vi "Main Monitor Loop.vi"(8 "error in (no error)":errorcluster, 11 "main ref":T1) -> (0 "error out":errorcluster)   [LabVIEW 2025]
uses:
  controls/LAB-IQ UI Data.ctl
  Traction Loop/Traction Receipe Enum.ctl
panel:
  out "Test Stop Temp":bool
  out "DepthZ":dbl
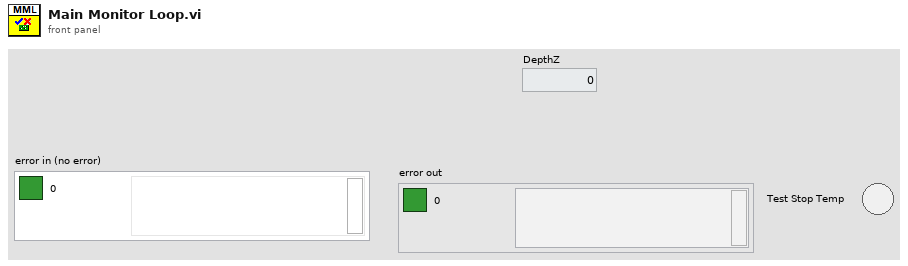
[diagram p1: front panel]
types:
  T1 = typedef "LAB-IQ UI Data.ctl" = cluster{"Main Home Screen":cluster{"GUI":refnum<vi>, "Platform Settings":refnum<vi>, "Configure":refnum<vi>, "Home":refnum<vi>, "EXIT":refnum<vi>, "service 2":refnum<vi>, "MainPage":refnum<vi>, "Analysis":refnum<vi>}, "Platform Settings":cluster{"mm/s  Surge":refnum<vi>, "Update Surge Speed":refnum<vi>, "Drive Error":refnum<vi>, "Disable Axis Jog Soft Limits":refnum<vi>, "mm/s  Sway":refnum<vi>, "Sway and Surge COM Status":refnum<vi>, "Heave COM Status":refnum<vi>, "Enable Platform":refnum<vi>, "Surge Forward Main":refnum<vi>, "Sway Right Main":refnum<vi>, "Sway Left Main":refnum<vi>, "Heave Down Main":refnum<vi>, "Heave Up main":refnum<vi>, "Update Sway Speed":refnum<vi>, "Update Heave Speed":refnum<vi>, "mm/s Heave":refnum<vi>, "mm/sec":refnum<vi>, "mm":refnum<vi>, "Surge Backward Main":refnum<vi>}, "Analysis Screen":cluster{"Analysis Home":refnum<vi>, "Surface Analysis":refnum<vi>, "Imaging":refnum<vi>, "Image Analysis":refnum<vi>, "Post Analysis":refnum<vi>}, "Config Screen":cluster{"Select Load Head":refnum<vi>, "Notes :":refnum<vi>, "FILE":refnum<vi>, "Sample ID :":refnum<vi>, "Operator ID :":refnum<vi>, "Operator Name :":refnum<vi>, "Auto":refnum<vi>}, "Motion Module":cluster{"zNL":refnum<vi>, "NL disp":refnum<vi>, "Rotary Tab":refnum<vi>, "Motion Direction:  3":refnum<vi>, "E.Velocity 2":refnum<vi>, "e.v/ssr 2":refnum<vi>, "Enter Fixed E.Velocity 2":refnum<vi>, "Enter Final SRR 2":refnum<vi>, "Enter initial SRR 2":refnum<vi>, "Enter Fixed SRR 2":refnum<vi>, "Enter the Final E.Velocity (m/s) 2":refnum<vi>, "Enter initial E.Velocity (m/s) 2":refnum<vi>, "Final Speed (RPM) 3":refnum<vi>, "Initial Speed (RPM) 2":refnum<vi>, "Enter the Final Velocity (m/s) 3":refnum<vi>, "Enter initial Velocity (m/s)  3":refnum<vi>, "Ramp Up 2":refnum<vi>, "TEST SELECTION":refnum<vi>, "SPEED SELECTION : ":refnum<vi>, "Angular Oscillation Set":refnum<vi>, "Traction":refnum<vi>, "Step Speed":refnum<vi>, "StepTable For Load-Speed":refnum<vi>, "StepTable For Speed":refnum<vi>, "Surge Forward MM":refnum<vi>, "Surge Backward MM":refnum<vi>, "M3 Image":refnum<vi>, "String 39":refnum<vi>, "Sway Left MM":refnum<vi>, "Sway Right MM":refnum<vi>, "Disable Axis Jog Soft Limits":refnum<vi>, "mm":refnum<vi>, "Heave Down MM":refnum<vi>, "Heave Up MM":refnum<vi>, "Wear Track Diameter (mm)":refnum<vi>, "Set WTD":refnum<vi>, "HomeScratch":refnum<vi>, "HomeRot":refnum<vi>, "PlaceModule":refnum<vi>, "Enter the Angle (Deg)":refnum<vi>, "Enter the Frequency (Hz)":refnum<vi>, "Motion Mode:":refnum<vi>, "LR Sway":refnum<vi>, "Rot Hor":refnum<vi>, "Scratch":refnum<vi>, "LR Cam":refnum<vi>, "MMBack":refnum<vi>, "MMNext":refnum<vi>, "Rot Ver":refnum<vi>, "Rotary Module Selection":refnum<vi>, "calculate rotary":refnum<vi>, "SPEED SELECTION : rotary":refnum<vi>, "Import 2":refnum<vi>, "Save 2":refnum<vi>, "File Path :  2":refnum<vi>, "String 45":refnum<vi>, "StepTable For Speed 3":refnum<vi>, "Enter the Speed(mm/sec)":refnum<vi>, "Enter the Speed(RPM)":refnum<vi>, "Enter Scratch Speed (mm/s):":refnum<vi>, "SwaySpeed Set":refnum<vi>, "Scartch Offset":refnum<vi>, "Motion type:":refnum<vi>, "HomeScratch 2":refnum<vi>, "Enter Scratch length (mm):":refnum<vi>, "Wear Track Diameter":refnum<vi>, "Rotary Speed Exced":refnum<vi>, "Scratch Mode":refnum<vi>, "No of Scratch":refnum<vi>}, "Environmental control":cluster{"Humidity  Status  3":refnum<vi>, "Low Temp  Status  2":refnum<vi>, "TK4 status 2":refnum<vi>, "Stage Temperature":refnum<vi>, "Sample Temperature":refnum<vi>, "Humidity (Amb)":refnum<vi>, "Clear List":refnum<vi>, "Add to list":refnum<vi>, "Wear":refnum<vi>, "Vibration":refnum<vi>, "Humidity (Chamber)":refnum<vi>, "Temperature (Chamber)":refnum<vi>, "ECR ":refnum<vi>, "Temperature (Amb)":refnum<vi>, "Microphone":refnum<vi>, "Acoustic Emission 3":refnum<vi>, "SNext":refnum<vi>, "APBack":refnum<vi>, "Enter the Temperature (°C):":refnum<vi>, "Enter the Stage \nTemperature (°C):":refnum<vi>, "Enter the Humidity (%Rh):":refnum<vi>, "Low Temp":refnum<vi>, "High Temp":refnum<vi>, "Humidity":refnum<vi>, "Sensors Picked":refnum<vi>}, "About Screen":cluster{"Password":refnum<vi>, "Home Service":refnum<vi>, "Advanced Setting":refnum<vi>, "About Tab":refnum<vi>, "ECR Port:":refnum<vi>, "Ramp Port:":refnum<vi>, "Installation/Replacement completed":refnum<vi>, "Loahead":refnum<vi>, "Heave and Surge COM Port:":refnum<vi>, "Sway COM Port:":refnum<vi>, "Temp Modbus:":refnum<vi>, "Humidity Port:":refnum<vi>, "Edit Gain Constants":refnum<vi>, "Save Gain Constants":refnum<vi>}, "Main Screen":cluster{"Main Screen Tab":refnum<vi>, "Angle and Frequency":refnum<vi>, "Stroke (mm)":refnum<vi>, "Angle (Deg)":refnum<vi>, "Main Speed Tab":refnum<vi>, "MTM MOTOR DISPLAY":refnum<vi>, "Disc Speed (m/sec)":refnum<vi>, "Ball Speed (m/sec)":refnum<vi>, "Disc Speed (RPM)":refnum<vi>, "Ball Speed (RPM)":refnum<vi>, "SPEED TAB":refnum<vi>, "Speed (m/sec)":refnum<vi>, "Set Speed (m/sec)":refnum<vi>, "Speed (RPM)":refnum<vi>, "Set Speed":refnum<vi>, "Time Tab":refnum<vi>, "Time ( HH:MM:SS ) 2":refnum<vi>, "Test Duration":refnum<vi>, "Test Duration 4":refnum<vi>, "TEST CYCLE":refnum<vi>, "TOTAL CYCLES":refnum<vi>, "Set Load (N)":refnum<vi>, "Temp Tabs":refnum<vi>, "Heater":refnum<vi>, "TK4 status":refnum<vi>, "ChamberTemp":refnum<vi>, "SetTmp":refnum<vi>, "Controller  Status":refnum<vi>, "ChamberTemp 2":refnum<vi>, "SetTmp 2":refnum<vi>, "Controller  Status 2":refnum<vi>, "ChamberTemp 3":refnum<vi>, "SetTmp 3":refnum<vi>, "Cooling":refnum<vi>, "Load Communication":refnum<vi>, "Ambient \nTemperature":refnum<vi>, "HumCOMStatus":refnum<vi>, "Ambient\n Humidity":refnum<vi>, "Freq (Hz)":refnum<vi>, "Load En":refnum<vi>, "NLt":refnum<vi>, "zNL 2":refnum<vi>, "Humidity On":refnum<vi>, "humidity disp":refnum<vi>, "Set Humidity":refnum<vi>, "NL disp 2":refnum<vi>, "Humidity On 2":refnum<vi>, "humidity disp 2":refnum<vi>, "Set Humidity 2":refnum<vi>, "NL disp 3":refnum<vi>, "AppLoadSeq scratch":refnum<vi>, "Stop Scratch":refnum<vi>, "ClrLog":refnum<vi>, "Trip Log":refnum<vi>, "STOP":refnum<vi>, "Start Test":refnum<vi>, "Test status":refnum<vi>, "AR Led":refnum<vi>, "Data":refnum<vi>, "Health":refnum<vi>, "Sway COM Status":refnum<vi>, "Heave COM Status":refnum<vi>, "Grp Tab":refnum<vi>, "Sub Graph":refnum<vi>, "SD (mm)":refnum<vi>, "Siliding distance Reset Graph":refnum<vi>, "SDGp":refnum<vi>, "Humidity Reset Graph":refnum<vi>, "HumrGp":refnum<vi>, "Acoustic Emission (mV)":refnum<vi>, "Aqucostic Reset Graph":refnum<vi>, "gACQUOS":refnum<vi>, "ECR RESET":refnum<vi>, "ECR":refnum<vi>, "Temperature Reset":refnum<vi>, "Acoustic Emission (mV) 2":refnum<vi>, "Aqucostic Reset Graph 2":refnum<vi>, "gACQUOS 2":refnum<vi>, "ECR RESET 2":refnum<vi>, "ECR 2":refnum<vi>, "Temperature Reset 2":refnum<vi>, "Temperature (deg c)":refnum<vi>, "Speed Reset Graph":refnum<vi>, "Speed Tab":refnum<vi>, "MTM DISC  SPEED":refnum<vi>, "MTM BALL SPEED":refnum<vi>, "speed mm/sec":refnum<vi>, "Hymidity":refnum<vi>, "Humidity Disable trip":refnum<vi>, "CoF Trip  2":refnum<vi>, "Depth Trip":refnum<vi>, "Weart Deapth":refnum<vi>, "Depth Reset Graph":refnum<vi>, "Weart":refnum<vi>, "Depthz":refnum<vi>, "Depth (µm)":refnum<vi>, "WearGp":refnum<vi>, "NL Trip 2":refnum<vi>, "Load pid":refnum<vi>, "Load Disable Trip":refnum<vi>, "Load Reset Graph":refnum<vi>, "NL Display 4":refnum<vi>, "Main Chart 3":refnum<vi>, "BACK":refnum<vi>, "Depth Trip 2":refnum<vi>, "COF TRIP ":refnum<vi>, "Friction Force (N)":refnum<vi>, "FF Reset Graph":refnum<vi>, "FF Disable Trip":refnum<vi>, "FF TRIP":refnum<vi>, "COF Disable Trip":refnum<vi>, "COF Reset Graph":refnum<vi>, "Start Test Temp":refnum<vi>, "zFF":refnum<vi>, "Friction Force (N) Graph":refnum<vi>, "Coefficient of Friction":refnum<vi>, "Scratch Start Test":refnum<vi>, "FF Tab":refnum<vi>, "Cyclic Friction Force (N)":refnum<vi>, "CZ FF":refnum<vi>, "Cyclic Friction Force (N) Graph":refnum<vi>, "Cyclic Coefficient of Friction":refnum<vi>, "Cyclic FF TRIP":refnum<vi>, "Cyclic FF Disable Trip":refnum<vi>, "cyclic COF Disable Trip":refnum<vi>, "cyclic COF TRIP":refnum<vi>, "cyclic COF Reset Graph":refnum<vi>, "Cyclic FF Reset Graph":refnum<vi>, "Test Trip":refnum<vi>, "Multi Scratch Pass":refnum<vi>, "Scratch Start Recording":refnum<vi>}, "Loading":cluster{"Indentation":refnum<vi>, "Reference Sample":refnum<vi>, "Load Cell Communication Slide":refnum<vi>, "com 3":refnum<vi>, "com":refnum<vi>, "DecaForce COM Status":refnum<vi>, "Update":refnum<vi>, "Clear 3":refnum<vi>, "seq":refnum<vi>, "Stribeck table":refnum<vi>, "Stribeck Table  For loading":refnum<vi>, "Loading Mode":refnum<vi>, "Enter the Final Load (N)":refnum<vi>, "Enter the CoF Trip":refnum<vi>, "Enter the Friction Force Trip":refnum<vi>, "Enter the Normal load Trip":refnum<vi>, "Enter the Load  (N)":refnum<vi>, "KiloForce":refnum<vi>, "DecaForce ":refnum<vi>, "MicroForce":refnum<vi>, "LHBack":refnum<vi>, "LHNext":refnum<vi>, "Enter the Loading Rate (N/min)":refnum<vi>, "Message":refnum<vi>, "Warning 2":refnum<vi>, "SSP 0.75":refnum<vi>, "SSP 0.5":refnum<vi>, "SSP 0.3":refnum<vi>, "Warning":refnum<vi>, "gui GIF":refnum<vi>, "Communication is established":refnum<vi>, "AppLoad 4":refnum<vi>, "Multipoint":refnum<vi>, "Load Selection":refnum<vi>}, "PID":cluster{"Ramp MulFac":refnum<vi>, "pulses LoadDiffRamp(2..10)":refnum<vi>, "PulseControlRamp(diff<=3N)":refnum<vi>, "SetLoadDeadband(%) Load(0-10N)":refnum<vi>, "PID gains out delay (microForce)":refnum<vi>, "Ramp":refnum<vi>, "Gain 2":refnum<vi>, "pulses LoadDiff(2..10)":refnum<vi>, "pulses LoadDiff(11..50)":refnum<vi>, "PulseControl(diff<=3N)":refnum<vi>, "SetLoadDeadband(%)  2":refnum<vi>, "Dummy Run":refnum<vi>, "Vertical load (N)":refnum<vi>, "AutoTune":refnum<vi>, "Offset 3 ":refnum<vi>, "apply load":refnum<vi>, "Offset  3":refnum<vi>, "apply load 2":refnum<vi>, "Enter ByPass Load":refnum<vi>, "reinit 3":refnum<vi>, "output range delay":refnum<vi>, "PID gains out delay":refnum<vi>, "Bypass Load":refnum<vi>, "pulsesSent":refnum<vi>, "pulses ":refnum<vi>, "actpid":refnum<vi>, "gFF Rot":refnum<vi>, "pulses LoadDiff(21..1000)":refnum<vi>, "Delay":refnum<vi>, "deadband":refnum<vi>}, "Config Parameters":cluster{"Tab Control 3":refnum<vi>, "Tab Control 19":refnum<vi>, "SAMPLES":refnum<vi>, "Re-initilaize":refnum<vi>, "Filter ON/OFF":refnum<vi>, "TracHomeSurgeOffsetCounts 10MM":refnum<vi>, "TracHomeSwayOffsetCounts 10MM":refnum<vi>, "Acoustic Emission:":refnum<vi>, "Apply Filter (FF)":refnum<vi>, "Filter% 2":refnum<vi>, "Apply Filter (Load)":refnum<vi>, "Filter% ":refnum<vi>, "Sway distance (mm)":refnum<vi>, "Surge distance (mm)":refnum<vi>, "DataSavingLoopDelay(ms)":refnum<vi>, "SAVE 2":refnum<vi>, "Enter Distance":refnum<vi>, "Sway Counts:":refnum<vi>, "Distance (mm): 3":refnum<vi>, "Surge Counts:":refnum<vi>, "Distance (mm): 2":refnum<vi>, "Distance (mm):":refnum<vi>, "Heave Counts:":refnum<vi>, "LRMHomeSurgeOffsetCounts":refnum<vi>, "LRMHomeSwayOffsetCounts":refnum<vi>, "TracHomeSurgeOffsetCounts 20MM":refnum<vi>, "TracHomeSwayOffsetCounts 20MM":refnum<vi>, "RotHomeSwayOffsetCounts":refnum<vi>, "RotHomeSurgeOffsetCounts":refnum<vi>, "Heave distance":refnum<vi>, "Zmm":refnum<vi>, "Heave Pulses/mm":refnum<vi>, "Surge Pulses/mm":refnum<vi>, "Sway Pulses/mm":refnum<vi>, "Heave Pitch":refnum<vi>, "Surge Pitch":refnum<vi>, "Sway Pitch":refnum<vi>, "Heave PPR":refnum<vi>, "Surge PPR":refnum<vi>, "Sway PPR":refnum<vi>, "Tab Control 5":refnum<vi>, "Tab Control 14":refnum<vi>, "Tab Control 26":refnum<vi>, "AE":refnum<vi>, "Heave Loop Delay":refnum<vi>, "Heave PID Speed":refnum<vi>, "Surge Jog Speed":refnum<vi>, "Heave Jog Speed":refnum<vi>, "Sway Loop Delay":refnum<vi>, "Sway PID Speed":refnum<vi>, "Sway Jog Speed":refnum<vi>, "DEPTH TRIP VALUE":refnum<vi>, "LOAD TRIP VALUE":refnum<vi>, "DEPTH TRIP   ENABLE":refnum<vi>, "LOAD TRIP  ENABLE":refnum<vi>, "CYCLIC FF TRIP VALUE":refnum<vi>, "FF TRIP VALUE":refnum<vi>, "CYCLIC CoF TRIP VALUE":refnum<vi>, "COF TRIP VALUE":refnum<vi>, "CYCLIC COF TRIP  ENABLE":refnum<vi>, "CYCLIC FF TRIP  ENABLE":refnum<vi>, "FF TRIP  ENABLE":refnum<vi>, "COF TRIP  ENABLE":refnum<vi>, "JOG TRIP LOAD VALUE (N)":refnum<vi>, "Rotary Vertical":refnum<vi>, "Traction":refnum<vi>, "Scratch":refnum<vi>, "LRM CAM":refnum<vi>, "Sway LRM":refnum<vi>, "Rotary Horizontal":refnum<vi>}, "Loading Com Port":cluster{"ClearAll":refnum<vi>, "Mz(Nm)":refnum<vi>, "My(Nm)":refnum<vi>, "Mx(Nm)":refnum<vi>, "Save Dwell":refnum<vi>, "Mx ":refnum<vi>, "My ":refnum<vi>, "Mz":refnum<vi>, "Fx(N)":refnum<vi>, "Fy(N)":refnum<vi>, "Fz(N)":refnum<vi>, "ZeroAll":refnum<vi>, "Acq Delay (ms)":refnum<vi>, "Burst Delay (ms)":refnum<vi>, "model":refnum<vi>, "SN":refnum<vi>, "FFx(N)":refnum<vi>, "Sensor IP":refnum<vi>, "Port":refnum<vi>, "FFy(N)":refnum<vi>, "Load(N)":refnum<vi>, "delete Handle":refnum<vi>, "Create Handle":refnum<vi>, "ft_data":refnum<vi>, "ft_range":refnum<vi>, "ft_data 2":refnum<vi>, "stop 6":refnum<vi>, "running_flag":refnum<vi>, "ft_udp_handle":refnum<vi>, "get-data-return":refnum<vi>, "get-range-return":refnum<vi>, "zero-return":refnum<vi>, "filter-return":refnum<vi>, "initial-return":refnum<vi>, "deleteHandle-result":refnum<vi>, "Load Cell Temp":refnum<vi>, "Load Cell":refnum<vi>}, "Heave AND Surge":cluster{"SURGE POSE":refnum<vi>, "error out Read":refnum<vi>, "HEAVE POSE":refnum<vi>, "State":refnum<vi>, "Homed":refnum<vi>, "Sequence ID":refnum<vi>, "error out Write":refnum<vi>, "faultCode":refnum<vi>, "Ack ID":refnum<vi>, "SPEED":refnum<vi>, "Distance":refnum<vi>, "Mode Command":refnum<vi>, "Heave and Surge Read":refnum<vi>, "Read Heave Temp":refnum<vi>, "Spare 15":refnum<vi>, "Spare 14":refnum<vi>, "Spare 13":refnum<vi>, "Spare 12":refnum<vi>, "Spare 11":refnum<vi>, "Spare 10":refnum<vi>, "Spare 9":refnum<vi>, "Spare 8":refnum<vi>, "Spare 7":refnum<vi>, "Spare 6":refnum<vi>, "Spare 5":refnum<vi>, "Spare 4":refnum<vi>, "Spare 2":refnum<vi>, "Spare 1":refnum<vi>, "Node Id":refnum<vi>, "Spare 3":refnum<vi>, "SPARE 4":refnum<vi>, "SPARE 3":refnum<vi>, "SPARE 2":refnum<vi>, "SPARE 1":refnum<vi>, "fwMajor":refnum<vi>, "fwMinor":refnum<vi>, "Manual Write":refnum<vi>, "Heave and Surge Write":refnum<vi>, "SPARE 5":refnum<vi>, "Reserved ":refnum<vi>, "SPARE 8":refnum<vi>, "SPARE 6":refnum<vi>, "SPARE 7":refnum<vi>, "SPARE 17":refnum<vi>, "SPARE 16":refnum<vi>, "SPARE 15":refnum<vi>, "SPARE 14":refnum<vi>, "SPARE 13":refnum<vi>, "SPARE 12":refnum<vi>, "SPARE 11":refnum<vi>, "SPARE 10":refnum<vi>, "SPARE 9":refnum<vi>, "System UPTIME":refnum<vi>, "Missed Packets":refnum<vi>, "faultCode Surge Right":refnum<vi>, "faultCode Surge Left":refnum<vi>, "faultCode Heave":refnum<vi>, "UPLINK HEAVE":refnum<vi>, "DOWNLINK HEAVE":refnum<vi>}, "New PID LOGIC":cluster{"Fine Tune Zone":refnum<vi>, "PID SDelay":refnum<vi>, "Max_pos_limit":refnum<vi>, "Min_pos_limit":refnum<vi>, "i_limit":refnum<vi>, "pct_scale":refnum<vi>, "Deadband":refnum<vi>, "Kd":refnum<vi>, "Ki":refnum<vi>, "Kp":refnum<vi>, "Current Position":refnum<vi>, "Set Load":refnum<vi>, "Current Load":refnum<vi>, "Pulse delta":refnum<vi>, "Init Step":refnum<vi>, "Max Step Linit":refnum<vi>, "min_deadband_floor":refnum<vi>, "dynamic_spindle_noise_scalar":refnum<vi>, "min_finetune_floor":refnum<vi>, "filter_alpha":refnum<vi>, "PID":refnum<vi>}, "SWAY ":cluster{"fwMajor":refnum<vi>, "Homed":refnum<vi>, "Rotary POSE":refnum<vi>, "State":refnum<vi>, "SWAY POSE":refnum<vi>, "Ack ID":refnum<vi>, "faultCode":refnum<vi>, "Node Id":refnum<vi>, "fwMinor":refnum<vi>, "Spare 6":refnum<vi>, "Spare 5":refnum<vi>, "Spare 4":refnum<vi>, "Spare 3":refnum<vi>, "Spare 2":refnum<vi>, "Spare 1":refnum<vi>, "Spare 7":refnum<vi>, "SPARE  5":refnum<vi>, "error out Write  SWAY ":refnum<vi>, "error out Read SWAY ":refnum<vi>, "Manual Write SWAY ":refnum<vi>, "SWAY WRITE":refnum<vi>, "SPARE  4":refnum<vi>, "SPARE  3":refnum<vi>, "SPARE 2":refnum<vi>, "SPARE 1":refnum<vi>, "Spare 15":refnum<vi>, "Spare 14":refnum<vi>, "Spare 13":refnum<vi>, "Spare 12":refnum<vi>, "Spare 11":refnum<vi>, "Spare 9":refnum<vi>, "Spare 8":refnum<vi>, "SPEED":refnum<vi>, "Distance":refnum<vi>, "Mode Command":refnum<vi>, "Sequence ID":refnum<vi>, "SWAY READ":refnum<vi>, "Spare 10":refnum<vi>, "Read SWAY Temp":refnum<vi>, "faultCode Sway ":refnum<vi>, "Missed Packets":refnum<vi>, "System UPTIME sway":refnum<vi>, "SPARE 6":refnum<vi>, "SPARE 7":refnum<vi>, "SPARE 9":refnum<vi>, "SPARE 11":refnum<vi>, "SPARE 10":refnum<vi>, "SPARE 8":refnum<vi>, "SPARE 13":refnum<vi>, "SPARE 12":refnum<vi>, "SPARE 17":refnum<vi>, "SPARE 16":refnum<vi>, "SPARE 15":refnum<vi>, "SPARE 14":refnum<vi>, "Reserved":refnum<vi>, "faultCode Rotary":refnum<vi>, "UPLINK SWAY":refnum<vi>, "DOWNLINK SWAY":refnum<vi>}, "Analysis Screen":cluster{"Analysis Home":refnum<vi>, "Refresh 2":refnum<vi>, "MEAN 4":refnum<vi>, "SD 4":refnum<vi>, "VARIANCE 4":refnum<vi>, "MEAN  3":refnum<vi>, "SD  3":refnum<vi>, "VARIANCE  3":refnum<vi>, "MEAN 2":refnum<vi>, "SD  2":refnum<vi>, "VARIANCE 2":refnum<vi>, "MEAN":refnum<vi>, "SD":refnum<vi>, "VARIANCE":refnum<vi>, "File 4 Discription":refnum<vi>, "OPEN 4":refnum<vi>, "File Name 4":refnum<vi>, "OPEN 3":refnum<vi>, "File 3 Discription":refnum<vi>, "File Name 3":refnum<vi>, "Y-AXIS":refnum<vi>, "X-AXIS":refnum<vi>, "XY Graph":refnum<vi>, "File Name 2":refnum<vi>, "File Name 1":refnum<vi>, "OPEN 2":refnum<vi>, "OPEN 1":refnum<vi>, "File 1 Discription ":refnum<vi>, "File 2 Discription":refnum<vi>, "Export":refnum<vi>, "File Format":refnum<vi>}, "Traction":cluster{"faultCode Traction 2":refnum<vi>, "faultCode Traction 1":refnum<vi>, "Missed Packets":refnum<vi>, "System UPTIME Traction":refnum<vi>, "SPARE 17":refnum<vi>, "SPARE 16":refnum<vi>, "SPARE 15":refnum<vi>, "SPARE 14":refnum<vi>, "SPARE 13":refnum<vi>, "SPARE 12":refnum<vi>, "SPARE 11":refnum<vi>, "SPARE 10":refnum<vi>, "SPARE 9":refnum<vi>, "SPARE 8":refnum<vi>, "SPARE 7":refnum<vi>, "SPARE 6":refnum<vi>, "Reserved":refnum<vi>, "SPARE  5":refnum<vi>, "Manual Write TRACTION":refnum<vi>, "TRACTION WRITE":refnum<vi>, "SPARE  4":refnum<vi>, "SPARE  3":refnum<vi>, "SPARE 2":refnum<vi>, "SPARE 1":refnum<vi>, "Spare 7":refnum<vi>, "Spare 6":refnum<vi>, "Spare 5":refnum<vi>, "Spare 4":refnum<vi>, "Spare 2":refnum<vi>, "Spare 1":refnum<vi>, "Node Id":refnum<vi>, "Read TRACTION Temp":refnum<vi>, "fwMinor":refnum<vi>, "fwMajor":refnum<vi>, "faultCode":refnum<vi>, "TRACTION POSE":refnum<vi>, "TRACTION POSE 2":refnum<vi>, "Homed":refnum<vi>, "State":refnum<vi>, "Ack ID":refnum<vi>, "SPEED":refnum<vi>, "Distance":refnum<vi>, "Mode Command":refnum<vi>, "Sequence ID":refnum<vi>, "error out Read TRACTION":refnum<vi>, "error out Write  TRACTION":refnum<vi>, "TRACTION READ":refnum<vi>, "Spare 3":refnum<vi>, "Downlink traction":refnum<vi>, "Uplink Traction":refnum<vi>}, "Traction reciepe":cluster{"SRR Sweep Range (%) Stribeck":refnum<vi>, "Traction Receipe":refnum<vi>, "Total Execution Time":refnum<vi>, "Total Steps":refnum<vi>, "Duration / Step (s)  Stribeck":refnum<vi>, "STRIBECK Fixed SRR List (%)":refnum<vi>, "Duration / Step (s) Traction":refnum<vi>, "SRR Sweep Range (%) traction":refnum<vi>, "Rolling Speed (mm/s)":refnum<vi>, "Temperature Stages (°C)":refnum<vi>, "Ball Load (N)":refnum<vi>, "Lubricant Name":refnum<vi>, "Profile File Name":refnum<vi>, "SET entrainment Velocity":refnum<vi>, "Test Array Size":refnum<vi>, "SRR INDEX [ STRIBECK]":refnum<vi>, "Stribeck Size":refnum<vi>, "SET SRR":refnum<vi>, "ELAPSED TIMER ":refnum<vi>, "BALL SET RPM":refnum<vi>, "DISC SET RPM":refnum<vi>, "SET LOAD":refnum<vi>, "TEMPERATURE READ":refnum<vi>, "SET TEMPERATURE":refnum<vi>, "Traction Size":refnum<vi>, "DISC SPEED (rpm)":refnum<vi>, "BALL SPEED (rpm)":refnum<vi>, "BALL WEAR TRACK":refnum<vi>, "DISC WEARTRACK":refnum<vi>, "SRR INDEX [ TRACTION]":refnum<vi>, "Start Index Type":refnum<vi>, "Enum - Menu":refnum<vi>, "Ball (mm/sec)":refnum<vi>, "Disc (mm/sec)":refnum<vi>}, "Traction Control":cluster{"HomeTraction":refnum<vi>, "Demo Mode Display":refnum<vi>, "Traction Message":refnum<vi>, "Traction Step Update Details":refnum<vi>, "Main Tab sequence for selection":refnum<vi>, "Ramp Tab":refnum<vi>, "e.v/ssr":refnum<vi>, "Enter Fixed E.Velocity":refnum<vi>, "Enter Final SRR":refnum<vi>, "Enter initial SRR":refnum<vi>, "Enter Fixed SRR":refnum<vi>, "Enter the Final E.Velocity (m/s)":refnum<vi>, "Enter initial E.Velocity (m/s)":refnum<vi>, "Ball WTD":refnum<vi>, "E.Velocity":refnum<vi>, "Enter the Final Velocity (m/s)":refnum<vi>, "Enter initial Velocity (m/s)":refnum<vi>, "Ramp Up   Disc":refnum<vi>, "Initial DiscSpeed (RPM)":refnum<vi>, "Final Speed (RPM) Ball":refnum<vi>, "Final Speed (RPM)":refnum<vi>, "Initial Speed (RPM) Ball":refnum<vi>, "Enter the Final Velocity (m/s) Ball":refnum<vi>, "Enter initial Velocity (m/s) Ball":refnum<vi>, "Ramp Up":refnum<vi>, "ExceedBallSpeed step":refnum<vi>, "ExceedDiscSpeed":refnum<vi>, "BallSpeed Exceed Indication":refnum<vi>, "Apply":refnum<vi>, "SPEED SELECTION : MTM":refnum<vi>, "SPEED SELECTION : MTM 2":refnum<vi>, "TEST SELECTION (MTM)":refnum<vi>, "MTM Test Selection":refnum<vi>, "File Path Tab":refnum<vi>, "File Path String":refnum<vi>, "Save":refnum<vi>, "Save  2":refnum<vi>, "Import ":refnum<vi>, "File Path :":refnum<vi>, "Step Sequence Indication Tab":refnum<vi>, "Step Sequence Indication":refnum<vi>, "Calculate Step":refnum<vi>, "StepTable":refnum<vi>, "ExceedDiscSpeed  Cinstant Speed":refnum<vi>, "ExceedBallSpeed Constant":refnum<vi>, "TEST SELECTION (MTM) 2":refnum<vi>, "SPEED SELECTION : MTM 3":refnum<vi>, "MTM Test Selection 2":refnum<vi>, "Enter the Speed (m/sec): ":refnum<vi>, "Enter the Speed (m/sec):  2":refnum<vi>, "Enter the Speed (RPM):":refnum<vi>, "Lower Spped ":refnum<vi>, "Upper":refnum<vi>, "Enter the Speed (RPM):Ball":refnum<vi>, "Disc Motion Direction: ":refnum<vi>, "Ball Motion Direction :":refnum<vi>, "Motion Mode: ":refnum<vi>, "Wear Track Diameter (mm) ":refnum<vi>, "Disc Speed Indicator":refnum<vi>, "ExceedBallSpeed":refnum<vi>}, "Acquostic":cluster{"Last Config Rejected ":refnum<vi>, "rx command count":refnum<vi>, "Current Filter Id":refnum<vi>, "Isolated Gain":refnum<vi>, "DAQ Status":refnum<vi>, "error out":refnum<vi>, "error in (no error)":refnum<vi>, "Uplink Packet":refnum<vi>, "data out":refnum<vi>, "Downlink Packet":refnum<vi>, "Signal Energy":refnum<vi>, "Amplitude db_AE":refnum<vi>, "Peak Amplitude":refnum<vi>, "AE Ring-Down Counts":refnum<vi>, "Gains":refnum<vi>, "Manual Write Acquostic":refnum<vi>}}
  T2 = cluster{"Ack ID":u16, "State":u8, "Homed":u8, "HEAVE POSE":sgl, "SURGE POSE":sgl, "faultCode":u16, "fwMajor":u8, "fwMinor":u8, "Node Id":u8, "Spare 1":u8, "Spare 2":u8, "Spare 3":u8, "Spare 4":u8, "Spare 5":u8, "Spare 6":u8, "Spare 7":u8, "System UPTIME":sgl, "Missed Packets":sgl, "faultCode Heave":u16, "faultCode Surge Left":u16, "faultCode Surge Right":u16}
  T3 = cluster{"Ack ID ":u16, "State":u8, "Homed":u8, "SWAY POSE ":sgl, "Rotary POSE ":sgl, "faultCode":u16, "fwMajor":u8, "fwMinor":u8, "Node Id":u8, "Spare 1":u8, "Spare 2":u8, "Spare 3":u8, "Spare 4":u8, "Spare 5":u8, "Spare 6":u8, "Spare 7":u8, "System UPTIME ":sgl, "Missed Packets ":sgl, "faultCode Sway":u16, "faultCode Rotary":u16}
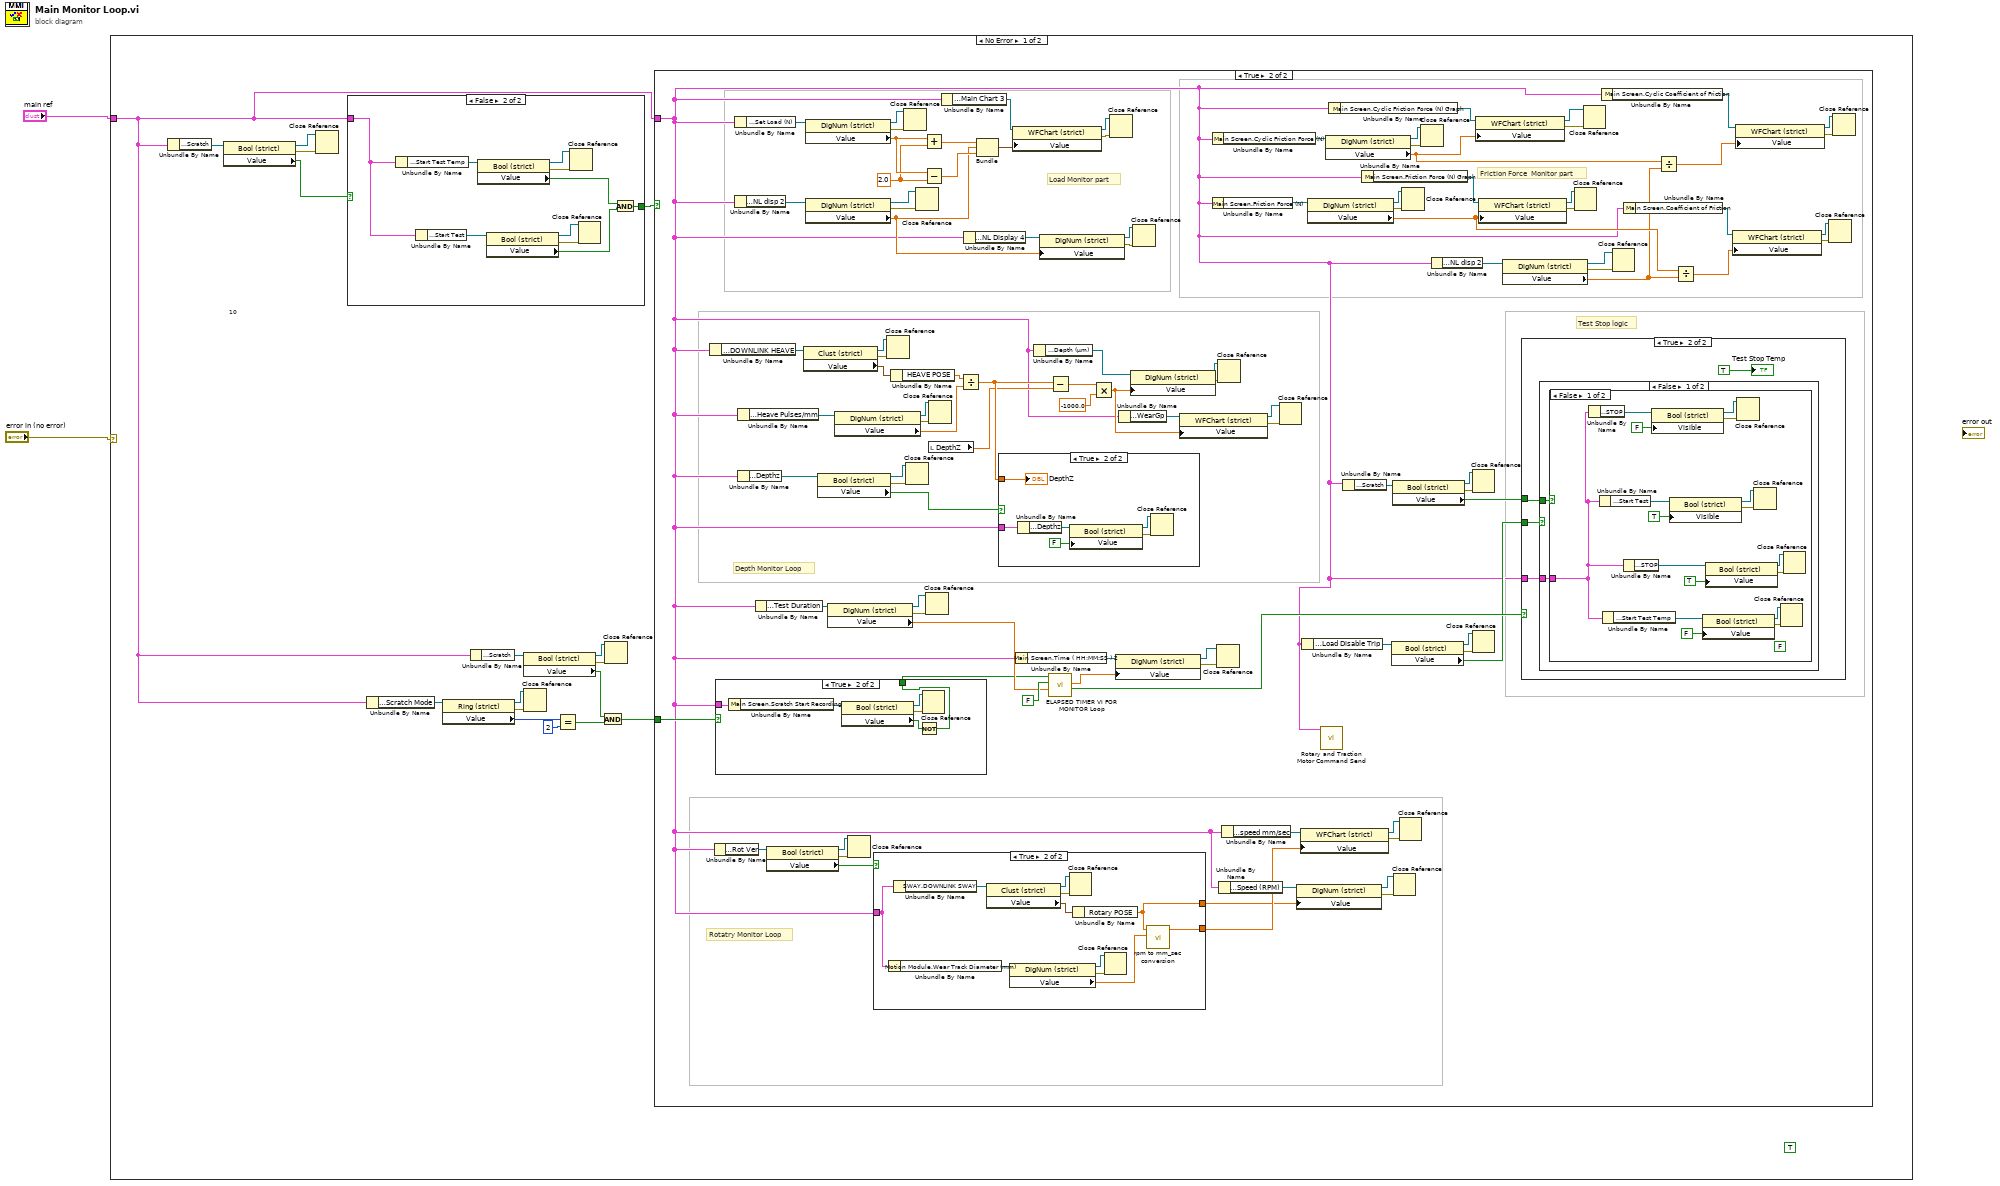
[diagram p0: block diagram]
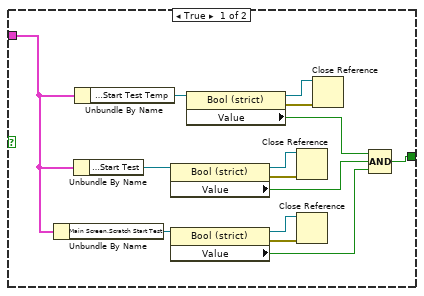
[diagram p2: hidden frame]
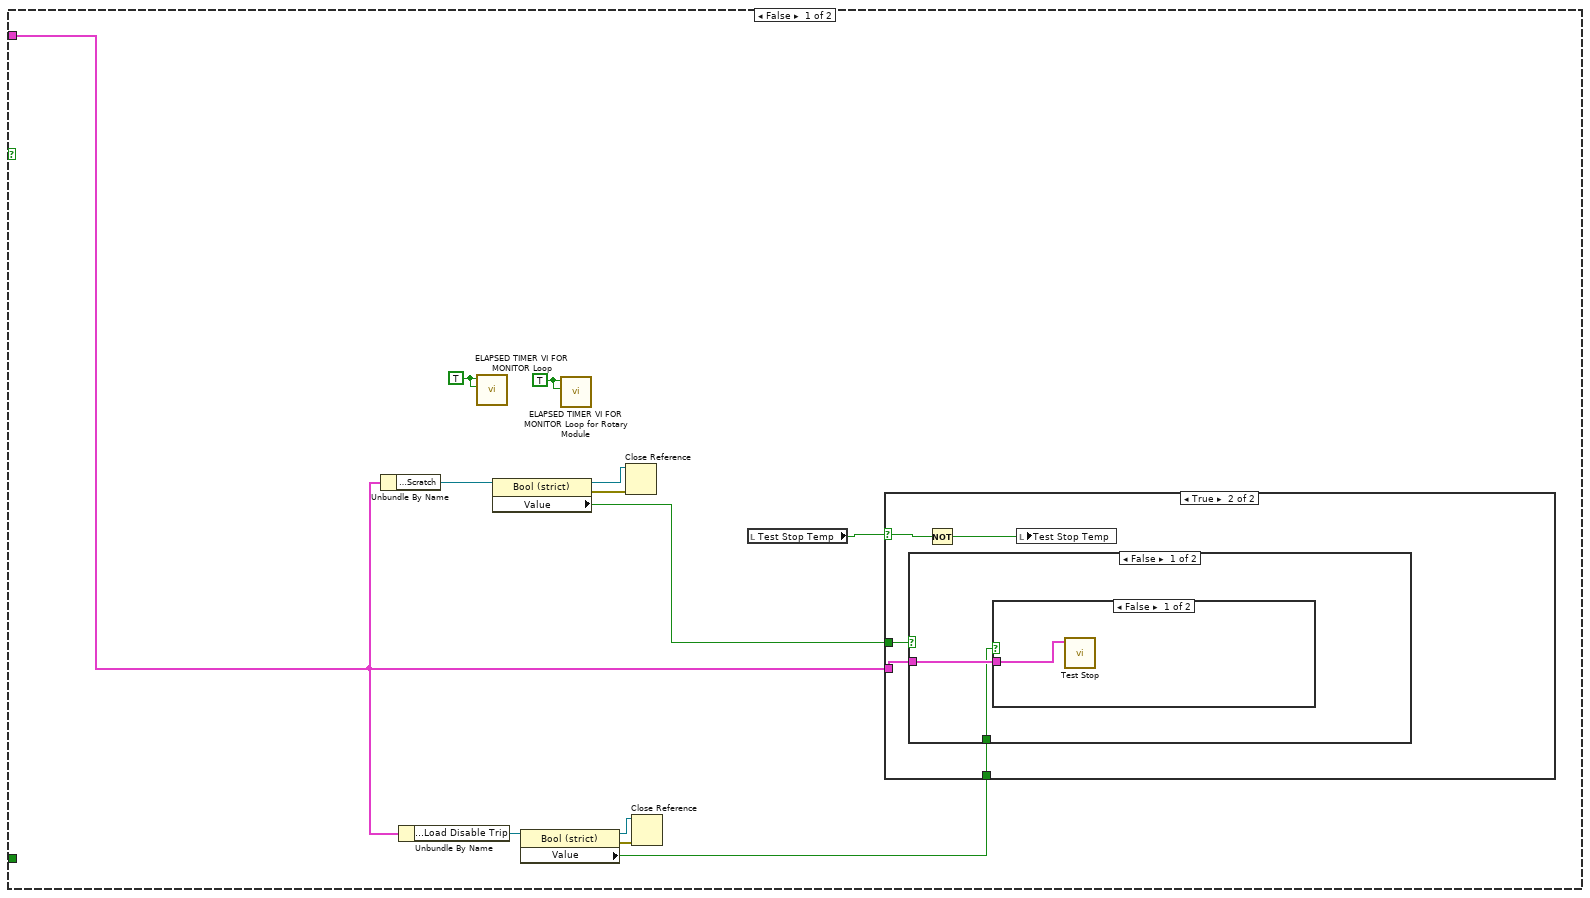
[diagram p3: hidden frame]
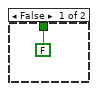
[diagram p7: hidden frame]
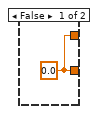
[diagram p8: hidden frame]
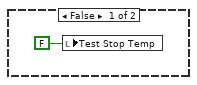
[diagram p9: hidden frame]
diagram:
  n1 = case shown="No Error" "error in (no error)" {
    tunnel: "main ref" -> [w6 _]
    frame No Error {
      (unwired) TRUE
      # "10"
      n2 = Unbundle By Name(w6) -> ("Motion Module.Scratch"=w17:refnum<vi>)
      n3 = property class="Bool (strict)"(reference=w17) -> (reference out=w18:refnum<vi>, error out=w16:errorcluster, "Value"=w15:bool)  [unwired: 1 in]
      n4 = Close Reference(reference=w18, error in (no error)=w16) -> ()  [unwired: 1 out]
      n5 = case shown="False" w15 {
        tunnel: w6 -> [w21 w37]
        tunnel: [w25 w35] -> w19
        frame True {
          n6 = Unbundle By Name(w21) -> ("Main Screen.Scratch Start Test"=w23:refnum<vi>)
          n7 = Unbundle By Name(w21) -> ("Main Screen.Start Test"=w29:refnum<vi>)
          n8 = Unbundle By Name(w21) -> ("Main Screen.Start Test Temp"=w32:refnum<vi>)
          n9 = property class="Bool (strict)"(reference=w29) -> (reference out=w28:refnum<vi>, error out=w30:errorcluster, "Value"=w26:bool)  [unwired: 1 in]
          n10 = property class="Bool (strict)"(reference=w23) -> (reference out=w24:refnum<vi>, error out=w22:errorcluster, "Value"=w20:bool)  [unwired: 1 in]
          n11 = property class="Bool (strict)"(reference=w32) -> (reference out=w33:refnum<vi>, error out=w31:errorcluster, "Value"=w27:bool)  [unwired: 1 in]
          n12 = Close Reference(reference=w28, error in (no error)=w30) -> ()  [unwired: 1 out]
          n13 = Close Reference(reference=w24, error in (no error)=w22) -> ()  [unwired: 1 out]
          n14 = Close Reference(reference=w33, error in (no error)=w31) -> ()  [unwired: 1 out]
          n15 = Compound Arithmetic op=AND(w27, w26, w20) -> (w25:bool)
        }
        frame False {
          n16 = Unbundle By Name(w37) -> ("Main Screen.Start Test Temp"=w42:refnum<vi>)
          n17 = Unbundle By Name(w37) -> ("Main Screen.Start Test"=w39:refnum<vi>)
          n18 = property class="Bool (strict)"(reference=w42) -> (reference out=w43:refnum<vi>, error out=w41:errorcluster, "Value"=w36:bool)  [unwired: 1 in]
          n19 = property class="Bool (strict)"(reference=w39) -> (reference out=w38:refnum<vi>, error out=w40:errorcluster, "Value"=w34:bool)  [unwired: 1 in]
          n20 = Close Reference(reference=w43, error in (no error)=w41) -> ()  [unwired: 1 out]
          n21 = Close Reference(reference=w38, error in (no error)=w40) -> ()  [unwired: 1 out]
          n22 = And(x=w36, y=w34) -> (x .and. y?=w35:bool)
        }
      }
      n23 = Unbundle By Name(w6) -> ("Motion Module.Scratch Mode"=w10:refnum<vi>)
      n24 = property class="Ring (strict)"(reference=w10) -> (reference out=w11:refnum<vi>, error out=w9:errorcluster, "Value"=w8:u16)  [unwired: 1 in]
      n25 = Unbundle By Name(w6) -> ("Motion Module.Scratch"=w13:refnum<vi>)
      n26 = property class="Bool (strict)"(reference=w13) -> (reference out=w12:refnum<vi>, error out=w14:errorcluster, "Value"=w4:bool)  [unwired: 1 in]
      n27 = Close Reference(reference=w11, error in (no error)=w9) -> ()  [unwired: 1 out]
      n28 = Equal?(x=w8, y=u16 2) -> (x = y?=w5:bool)
      n29 = And(x=w4, y=w5) -> (x .and. y?=w3:bool)
      n30 = Close Reference(reference=w12, error in (no error)=w14) -> ()  [unwired: 1 out]
      n31 = case shown="True" w19 {
        tunnel: w6 -> [w46 w64]
        tunnel: w3 -> [_ w71]
        frame False {
          w44 = TRUE ("PAUSE")
          w55 = TRUE ("PAUSE")
          n32 = Unbundle By Name(w46) -> ("Motion Module.Scratch"=w53:refnum<vi>)
          n33 = Unbundle By Name(w46) -> ("Main Screen.Load Disable Trip"=w47:refnum<vi>)
          n34 = call "ELAPSED TIMER VI FOR MONITOR Loop.vi"("RESET"=w55, "PAUSE"=w55) -> ()  [unwired: 7 in, 3 out]
          n35 = property class="Bool (strict)"(reference=w53) -> (reference out=w51:refnum<vi>, error out=w52:errorcluster, "Value"=w50:bool)  [unwired: 1 in]
          n36 = property class="Bool (strict)"(reference=w47) -> (reference out=w49:refnum<vi>, error out=w48:errorcluster, "Value"=w45:bool)  [unwired: 1 in]
          n37 = call "ELAPSED TIMER VI FOR MONITOR Loop for Rotary Module.vi"("RESET"=w44, "PAUSE"=w44) -> ()  [unwired: 7 in, 3 out]
          n38 = Close Reference(reference=w51, error in (no error)=w52) -> ()  [unwired: 1 out]
          n39 = Close Reference(reference=w49, error in (no error)=w48) -> ()  [unwired: 1 out]
          n40 = local read "Test Stop Temp"() -> (w54:bool)
          n41 = case shown="True" w54 {
            selector: w54 -> [_ w60]
            tunnel: w46 -> [_ w58]
            tunnel: w50 -> [_ w57]
            tunnel: w45 -> [_ w56]
            frame False {
            }
            frame True {
              n42 = case shown="False" w57 {
                tunnel: w58 -> [w62 _]
                tunnel: w56 -> [w61 _]
                frame False {
                  n43 = case shown="False" w61 {
                    tunnel: w62 -> [w63 _]
                    frame False {
                      n44 = call "Test Stop.vi"("Data Cluster"=w63) -> ()  [unwired: 10 in, 1 out]
                    }
                    frame True {
                    }
                  }
                }
                frame True {
                }
              }
              n45 = Not(x=w60) -> (.not. x?=w59:bool)
              n46 = local write "Test Stop Temp"(w59) -> ()
            }
          }
        }
        frame True {
          w152 = 2.0 ("y")
          # "Rotatry Monitor Loop"
          # "Test Stop logic"
          # "Depth Monitor Loop"
          # "Friction Force  Monitor part"
          # "Load Monitor part"
          n47 = Unbundle By Name(w64) -> ("Heave AND Surge.DOWNLINK HEAVE"=w67:refnum<vi>)
          n48 = Unbundle By Name(w64) -> ("Motion Module.Rot Ver"=w87:refnum<vi>)
          n49 = case shown="True" w71 {
            tunnel: w64 -> [_ w168]
            tunnel: [FALSE ("Value") w166] -> w70
            frame False {
            }
            frame True {
              n50 = Unbundle By Name(w168) -> ("Main Screen.Scratch Start Recording"=w170:refnum<vi>)
              n51 = property class="Bool (strict)"(reference=w170) -> (reference out=w169:refnum<vi>, error out=w171:errorcluster, "Value"=w167:bool)  [unwired: 1 in]
              n52 = Not(x=w167) -> (.not. x?=w166:bool)
              n53 = Close Reference(reference=w169, error in (no error)=w171) -> ()  [unwired: 1 out]
            }
          }
          n54 = Unbundle By Name(w64) -> ("Main Screen.Set Load (N)"=w154:refnum<vi>)
          n55 = Unbundle By Name(w64) -> ("Main Screen.NL disp 2"=w164:refnum<vi>)
          n56 = Unbundle By Name(w64) -> ("Config Parameters.Heave Pulses/mm"=w146:refnum<vi>)
          n57 = Unbundle By Name(w64) -> ("Main Screen.Depthz"=w142:refnum<vi>)
          n58 = Unbundle By Name(w64) -> ("Main Screen.Test Duration"=w126:refnum<vi>)
          n59 = property class="Bool (strict)"(reference=w87) -> (reference out=w85:refnum<vi>, error out=w86:errorcluster, "Value"=w84:bool)  [unwired: 1 in]
          n60 = property on="Property Node" class="Clust (strict)"(reference=w67) -> (reference out=w69:refnum<vi>, error out=w68:errorcluster, "Value"=w66:T2)  [unwired: 1 in]
          n61 = property class="DigNum (strict)"(reference=w154) -> (reference out=w148:refnum<vi>, error out=w155:errorcluster, "Value"=w153:dbl)  [unwired: 1 in]
          n62 = property class="DigNum (strict)"(reference=w164) -> (reference out=w162:refnum<vi>, error out=w163:errorcluster, "Value"=w103:dbl)  [unwired: 1 in]
          n63 = property class="Bool (strict)"(reference=w142) -> (reference out=w143:refnum<vi>, error out=w141:errorcluster, "Value"=w140:bool)  [unwired: 1 in]
          n64 = property class="DigNum (strict)"(reference=w126) -> (reference out=w127:refnum<vi>, error out=w125:errorcluster, "Value"=w124:dbl)  [unwired: 1 in]
          n65 = property class="DigNum (strict)"(reference=w146) -> (reference out=w145:refnum<vi>, error out=w147:errorcluster, "Value"=w144:dbl)  [unwired: 1 in]
          n66 = Close Reference(reference=w85, error in (no error)=w86) -> ()  [unwired: 1 out]
          n67 = case shown="True" w84 {
            tunnel: w64 -> [_ w174]
            tunnel: [w172 w179] -> w80
            tunnel: [w172 w173] -> w76
            frame False {
              w172 = 0.0 ("Enter initial Velocity (m/s)  4")
            }
            frame True {
              n68 = Unbundle By Name(w174) -> ("Motion Module.Wear Track Diameter (mm)"=w183:refnum<vi>)
              n69 = Unbundle By Name(w174) -> ("SWAY.DOWNLINK SWAY"=w176:refnum<vi>)
              n70 = property on="Property Node" class="Clust (strict)"(reference=w176) -> (reference out=w178:refnum<vi>, error out=w177:errorcluster, "Value"=w175:T3)  [unwired: 1 in]
              n71 = property class="DigNum (strict)"(reference=w183) -> (reference out=w181:refnum<vi>, error out=w182:errorcluster, "Value"=w180:dbl)  [unwired: 1 in]
              n72 = Close Reference(reference=w178, error in (no error)=w177) -> ()  [unwired: 1 out]
              n73 = Unbundle By Name(w175) -> ("Rotary POSE"=w173:sgl)
              n74 = Close Reference(reference=w181, error in (no error)=w182) -> ()  [unwired: 1 out]
              n75 = call "rpm to mm_sec conversion.vi"("Wear Track Diameter"=w180, "Initial Speed (RPM)"=w173) -> ("Enter initial Velocity (m/s)  4"=w179:dbl)  [unwired: 7 in, 2 out]
            }
          }
          n76 = Close Reference(reference=w69, error in (no error)=w68) -> ()  [unwired: 1 out]
          n77 = Unbundle By Name(w66) -> ("HEAVE POSE"=w65:sgl)
          n78 = Close Reference(reference=w148, error in (no error)=w155) -> ()  [unwired: 1 out]
          n79 = Close Reference(reference=w143, error in (no error)=w141) -> ()  [unwired: 1 out]
          n80 = Close Reference(reference=w162, error in (no error)=w163) -> ()  [unwired: 1 out]
          n81 = Add(x=w153, y=w152) -> (x+y=w151:dbl)
          n82 = Subtract(x=w153, y=w152) -> (x-y=w150:dbl)
          n83 = Close Reference(reference=w127, error in (no error)=w125) -> ()  [unwired: 1 out]
          n84 = Close Reference(reference=w145, error in (no error)=w147) -> ()  [unwired: 1 out]
          n85 = local read "DepthZ"() -> (w138:dbl)
          n86 = Unbundle By Name(w64) -> ("Main Screen.Main Chart 3"=w158:refnum<vi>)
          n87 = Divide(x=w65, y=w144) -> (x/y=w139:dbl)
          n88 = Unbundle By Name(w64) -> ("Main Screen.NL Display 4"=w159:refnum<vi>)
          n89 = Bundle(w151, "Value"=w103, w150) -> (w149:cluster{dbl, "Value":dbl, dbl})  [unwired: 1 in]
          n90 = case shown="True" w140 {
            tunnel: w139 -> [_ w213]
            tunnel: w64 -> [_ w209]
            frame False {
            }
            frame True {
              n91 = Unbundle By Name(w209) -> ("Main Screen.Depthz"=w211:refnum<vi>)
              n92 = property class="Bool (strict)"(reference=w211, "Value"=FALSE) -> (reference out=w210:refnum<vi>, error out=w212:errorcluster)  [unwired: 1 in]
              n93 = Close Reference(reference=w210, error in (no error)=w212) -> ()  [unwired: 1 out]
              "DepthZ" <- w213
            }
          }
          n94 = property class="WFChart (strict)"(reference=w158, "Value"=w149) -> (reference out=w156:refnum<vi>, error out=w157:errorcluster)  [unwired: 1 in]
          n95 = Unbundle By Name(w64) -> ("Main Screen.Time ( HH:MM:SS ) 2"=w90:refnum<vi>)
          n96 = Unbundle By Name(w64) -> ("Main Screen.Depth (µm)"=w136:refnum<vi>)
          n97 = property class="DigNum (strict)"(reference=w159, "Value"=w103) -> (reference out=w161:refnum<vi>, error out=w160:errorcluster)  [unwired: 1 in]
          n98 = call "ELAPSED TIMER VI FOR MONITOR Loop.vi"("TARGET"=w124, "RESET"=FALSE ("PAUSE"), "PAUSE"=w70) -> ("ELAPSED INDICATION"=w111:bool, "ELAPSED TIMER"=w89:dbl)  [unwired: 6 in, 1 out]
          n99 = Subtract(x=w139, y=w138) -> (x-y=w130:dbl)
          n100 = Multiply(x=w130, y=-1000.0) -> (x*y=w131:dbl)
          n101 = Close Reference(reference=w156, error in (no error)=w157) -> ()  [unwired: 1 out]
          n102 = property class="DigNum (strict)"(reference=w90, "Value"=w89) -> (reference out=w122:refnum<vi>, error out=w123:errorcluster)  [unwired: 1 in]
          n103 = Unbundle By Name(w64) -> ("Main Screen.WearGp"=w133:refnum<vi>)
          n104 = property class="DigNum (strict)"(reference=w136, "Value"=w131) -> (reference out=w137:refnum<vi>, error out=w135:errorcluster)  [unwired: 1 in]
          n105 = Close Reference(reference=w161, error in (no error)=w160) -> ()  [unwired: 1 out]
          n106 = property class="WFChart (strict)"(reference=w133, "Value"=w131) -> (reference out=w134:refnum<vi>, error out=w132:errorcluster)  [unwired: 1 in]
          n107 = Unbundle By Name(w64) -> ("Main Screen.Cyclic Friction Force (N)"=w107:refnum<vi>)
          n108 = Unbundle By Name(w64) -> ("Main Screen.Friction Force (N)"=w120:refnum<vi>)
          n109 = Close Reference(reference=w122, error in (no error)=w123) -> ()  [unwired: 1 out]
          n110 = Close Reference(reference=w137, error in (no error)=w135) -> ()  [unwired: 1 out]
          n111 = Unbundle By Name(w64) -> ("Main Screen.Speed (RPM)"=w79:refnum<vi>)
          n112 = Unbundle By Name(w64) -> ("Main Screen.speed mm/sec"=w81:refnum<vi>)
          n113 = Close Reference(reference=w134, error in (no error)=w132) -> ()  [unwired: 1 out]
          n114 = property class="DigNum (strict)"(reference=w79, "Value"=w76) -> (reference out=w77:refnum<vi>, error out=w78:errorcluster)  [unwired: 1 in]
          n115 = property class="WFChart (strict)"(reference=w81, "Value"=w80) -> (reference out=w83:refnum<vi>, error out=w82:errorcluster)  [unwired: 1 in]
          n116 = Unbundle By Name(w64) -> ("Main Screen.Load Disable Trip"=w73:refnum<vi>)
          n117 = property class="DigNum (strict)"(reference=w120) -> (reference out=w121:refnum<vi>, error out=w119:errorcluster, "Value"=w113:dbl)  [unwired: 1 in]
          n118 = call "Rotary and Traction Motor Command Send.vi"("main ref"=w64) -> ()  [unwired: 10 in, 1 out]
          n119 = property class="DigNum (strict)"(reference=w107) -> (reference out=w105:refnum<vi>, error out=w106:errorcluster, "Value"=w104:dbl)  [unwired: 1 in]
          n120 = Unbundle By Name(w64) -> ("Main Screen.Cyclic Friction Force (N) Graph"=w110:refnum<vi>)
          n121 = Unbundle By Name(w64) -> ("Motion Module.Scratch"=w88:refnum<vi>)
          n122 = Unbundle By Name(w64) -> ("Main Screen.Friction Force (N) Graph"=w91:refnum<vi>)
          n123 = property class="Bool (strict)"(reference=w73) -> (reference out=w75:refnum<vi>, error out=w74:errorcluster, "Value"=w72:bool)  [unwired: 1 in]
          n124 = property class="Bool (strict)"(reference=w88) -> (reference out=w97:refnum<vi>, error out=w98:errorcluster, "Value"=w96:bool)  [unwired: 1 in]
          n125 = Close Reference(reference=w77, error in (no error)=w78) -> ()  [unwired: 1 out]
          n126 = Close Reference(reference=w83, error in (no error)=w82) -> ()  [unwired: 1 out]
          n127 = Close Reference(reference=w121, error in (no error)=w119) -> ()  [unwired: 1 out]
          n128 = Close Reference(reference=w105, error in (no error)=w106) -> ()  [unwired: 1 out]
          n129 = Unbundle By Name(w64) -> ("Main Screen.NL disp 2"=w95:refnum<vi>)
          n130 = Close Reference(reference=w97, error in (no error)=w98) -> ()  [unwired: 1 out]
          n131 = Close Reference(reference=w75, error in (no error)=w74) -> ()  [unwired: 1 out]
          n132 = property class="WFChart (strict)"(reference=w110, "Value"=w104) -> (reference out=w108:refnum<vi>, error out=w109:errorcluster)  [unwired: 1 in]
          n133 = property class="WFChart (strict)"(reference=w91, "Value"=w113) -> (reference out=w117:refnum<vi>, error out=w118:errorcluster)  [unwired: 1 in]
          n134 = property class="DigNum (strict)"(reference=w95) -> (reference out=w93:refnum<vi>, error out=w94:errorcluster, "Value"=w92:dbl)  [unwired: 1 in]
          n135 = case shown="True" w111 {
            tunnel: w64 -> [_ w187]
            tunnel: w96 -> [_ w186]
            tunnel: w72 -> [_ w185]
            frame False {
              n136 = local write "Test Stop Temp"(FALSE ("Test Stop Temp")) -> ()
            }
            frame True {
              n137 = case shown="False" w185 {
                tunnel: w187 -> [w190 _]
                tunnel: w186 -> [w189 _]
                frame False {
                  n138 = case shown="False" w189 {
                    tunnel: w190 -> [w191 _]
                    frame False {
                      (unwired) FALSE ("y")
                      n139 = Unbundle By Name(w191) -> ("Main Screen.STOP"=w197:refnum<vi>)
                      n140 = Unbundle By Name(w191) -> ("Main Screen.Start Test"=w194:refnum<vi>)
                      n141 = Unbundle By Name(w191) -> ("Main Screen.Start Test Temp"=w205:refnum<vi>)
                      n142 = Unbundle By Name(w191) -> ("Main Screen.STOP"=w204:refnum<vi>)
                      n143 = property class="Bool (strict)"(reference=w197, "Visible"=FALSE) -> (reference out=w199:refnum<vi>, error out=w198:errorcluster)  [unwired: 1 in]
                      n144 = property class="Bool (strict)"(reference=w194, "Visible"=TRUE) -> (reference out=w192:refnum<vi>, error out=w193:errorcluster)  [unwired: 1 in]
                      n145 = property class="Bool (strict)"(reference=w205, "Value"=FALSE) -> (reference out=w207:refnum<vi>, error out=w206:errorcluster)  [unwired: 1 in]
                      n146 = property class="Bool (strict)"(reference=w204, "Value"=TRUE) -> (reference out=w202:refnum<vi>, error out=w203:errorcluster)  [unwired: 1 in]
                      n147 = Close Reference(reference=w199, error in (no error)=w198) -> ()  [unwired: 1 out]
                      n148 = Close Reference(reference=w192, error in (no error)=w193) -> ()  [unwired: 1 out]
                      n149 = Close Reference(reference=w207, error in (no error)=w206) -> ()  [unwired: 1 out]
                      n150 = Close Reference(reference=w202, error in (no error)=w203) -> ()  [unwired: 1 out]
                    }
                    frame True {
                    }
                  }
                }
                frame True {
                }
              }
              "Test Stop Temp" <- TRUE ("Test Stop Temp")
            }
          }
          n151 = Close Reference(reference=w117, error in (no error)=w118) -> ()  [unwired: 1 out]
          n152 = Close Reference(reference=w108, error in (no error)=w109) -> ()  [unwired: 1 out]
          n153 = Unbundle By Name(w64) -> ("Main Screen.Cyclic Coefficient of Friction"=w101:refnum<vi>)
          n154 = Close Reference(reference=w93, error in (no error)=w94) -> ()  [unwired: 1 out]
          n155 = Unbundle By Name(w64) -> ("Main Screen.Coefficient of Friction"=w115:refnum<vi>)
          n156 = Divide(x=w104, y=w92) -> (x/y=w100:dbl)
          n157 = Divide(x=w113, y=w92) -> (x/y=w112:dbl)
          n158 = property class="WFChart (strict)"(reference=w115, "Value"=w112) -> (reference out=w116:refnum<vi>, error out=w114:errorcluster)  [unwired: 1 in]
          n159 = property class="WFChart (strict)"(reference=w101, "Value"=w100) -> (reference out=w99:refnum<vi>, error out=w102:errorcluster)  [unwired: 1 in]
          n160 = Close Reference(reference=w116, error in (no error)=w114) -> ()  [unwired: 1 out]
          n161 = Close Reference(reference=w99, error in (no error)=w102) -> ()  [unwired: 1 out]
        }
      }
    }
    frame Error {
    }
  }
